vi "PH_SSAC.Calc Time4Main.vi"(0 "i ref in":refnum<vi>, 5 "error in":errorcluster) -> (14 "i ref out":refnum<vi>, 17 "Time for Main [fs]":dbl[](array[numeric]), 19 "error out":errorcluster)   [LabVIEW 2014, in "PH_SSAC.lvlib"]
uses:
  PH_SSAC.lvlib
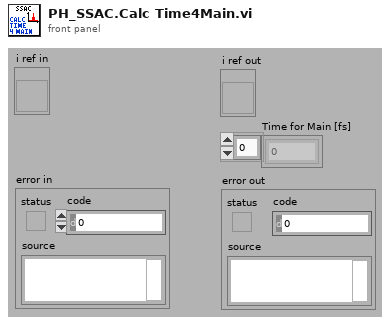
[diagram p1: front panel]
types:
  T1 = typedef "PH_SSAC.lvlib/PH_SSAC.i attribute.ctl" = cluster{"GUI Refs":cluster{"Delete":refnum<vi>, "Global On":refnum<vi>, "Cam Source":refnum<vi>, "Frame Main Signal":refnum<vi>, "Frame Background":refnum<vi>, "dt (Gauss smooth)":refnum<vi>, "Calibration Factor":refnum<vi>, "Background acquire":refnum<vi>, "Threshold":refnum<vi>, "Time evolution of mean pulse duration":refnum<vi>, "Mean Pulse Duration":refnum<vi>, "Main signal":refnum<vi>, "Current Pulse Duration":refnum<vi>, "Processed":refnum<vi>, "Saturation":refnum<vi>, "# for Average":refnum<vi>, "Position":refnum<vi>, "BG Status":refnum<vi>, "Save BG data":refnum<vi>, "Read BG Data":refnum<vi>, "Background Calibration Data":refnum<vi>}, "Images":cluster{"OP Image":T2, "GUI Image":T2, "PSDB Image":T2}, "Global On?":bool, "Frame Main":cluster{"x":u32, "dx":u32, "y":u32, "dy":u32}, "Frame Background":cluster{"x":u32, "dx":u32, "y":u32, "dy":u32}, "dt [fs]":dbl, "Calibration Factor [fs/pixel]":dbl, "Threshold":dbl, "Time evolution of mean pulse duration [fs]":dbl[], "Main Signal":cluster{"Time for Main":dbl[], "Signal":dbl[]}, "Processed":bool, "Current Pulse Duration [fs]":dbl, "# for Average":i32, "Position":i32, "Pulse Durations [fs]":dbl[], "BG":cluster{"Acquire?":bool, "Background Calibration Data":T3, "Save Data":bool}}
  T2 = typedef "IMAQ Image.ctl" = refnum<image>
  T3 = typedef "PH_SSAC.lvlib/PH_SSAC.Background Data.ctl" = cluster{"Date":string, "Time":string, "Frame Main":cluster{"x":u32, "dx":u32, "y":u32, "dy":u32}, "dt [fs]":dbl, "Calibration Factor [fs/pixel]":dbl, "Signal":dbl[], "Frame Background":cluster{"x":u32, "dx":u32, "y":u32, "dy":u32}}
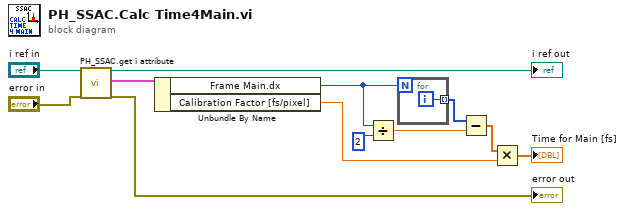
[diagram p0: block diagram]
diagram:
  n1 = call "PH_SSAC.get i attribute.vi"("i ref in"="i ref in", "error in (no error)"="error in") -> ("i ref out"=→"i ref out":refnum<vi>, "i attribute"=w10:T1, "error out"=→"error out":errorcluster)  [unwired: 15 in]
  n2 = Unbundle By Name(w10) -> ("Frame Main.dx"=w11:u32, "Calibration Factor [fs/pixel]"=w12:dbl)
  n3 = Divide(x=w11, y=2) -> (x/y=w3:dbl)
  n4 = for {
    N: w11 -> [_]
    tunnel: [w13] -> w2 mode=indexing
    i -> [w13]
  }
  n5 = Subtract(x=w2, y=w3) -> (x-y=w5:dbl[])
  n6 = Multiply(x=w5, y=w12) -> (x*y=→"Time for Main [fs]":dbl[])
